vi "simulation_testing.vi"() -> ()   [LabVIEW 2019]
panel:
  out "Waveform Chart":cluster{i16, i16}(graph)
  out "SDI":bool
  out "SCL":bool
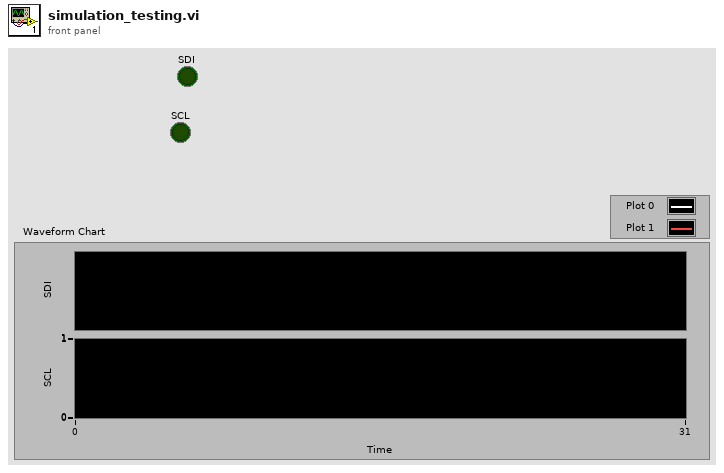
[diagram p1: front panel]
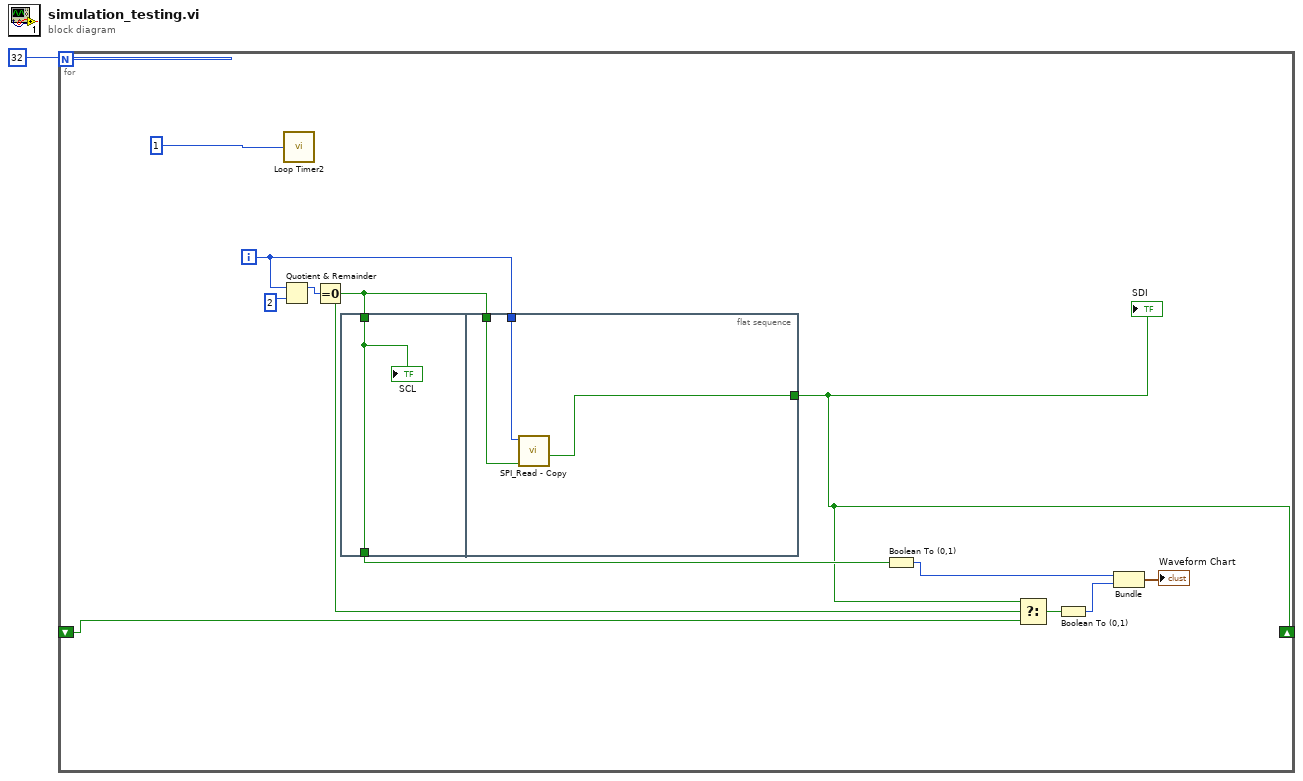
[diagram p0: block diagram]
diagram:
  n1 = for {
    N: 32 -> [_]
    shift-right: [w3] -> _
    shift-left: _ -> [w7]
    i -> [w10]
    n2 = Quotient & Remainder(x=w10, y=2) -> (x-y*floor(x/y)=w12:i32)  [unwired: 1 out]
    n3 = call "Loop Timer2"("Count(mSec)"=u32 1) -> ()  [unwired: 1 out]
    n4 = Equal To 0?(x=w12) -> (x = 0?=w9:bool)
    n5 = flat-sequence {
      tunnel: w9 -> [w14]
      tunnel: [w14] -> w8
      tunnel: w9 -> [w15]
      tunnel: w10 -> [w17]
      tunnel: [w16] -> w3
      frame #0 {
        "SCL" <- w14
      }
      frame #1 {
        n6 = call "SPI_Read - Copy.vi"("bit_index"=w17, "rising_edge"=w15) -> ("SDI"=w16:bool)  [unwired: 8 in]
      }
    }
    n7 = Boolean To (0,1)(Boolean=w8) -> (0, 1=w4:i16)
    n8 = Select(t=w3, s=w9, f=w7) -> (s? t:f=w6:bool)
    n9 = Boolean To (0,1)(Boolean=w6) -> (0, 1=w5:i16)
    n10 = Bundle(w4, w5) -> (→"Waveform Chart":cluster{i16, i16})  [unwired: 1 in]
    "SDI" <- w3
  }
